vi "Set All Front Panel Controls Disabled State.vi"(8 "error in (no error)":errorcluster, 10 "Disabled":T1(ring), 11 "Actor in":refnum<class "Actor.lvclass">) -> (0 "error out":errorcluster, 3 "Actor out":refnum<class "Actor.lvclass">)   [LabVIEW 2015, in "Actor.lvclass"]
uses:
  Actor.lvclass
  Actor.lvclass/Actor.ctl
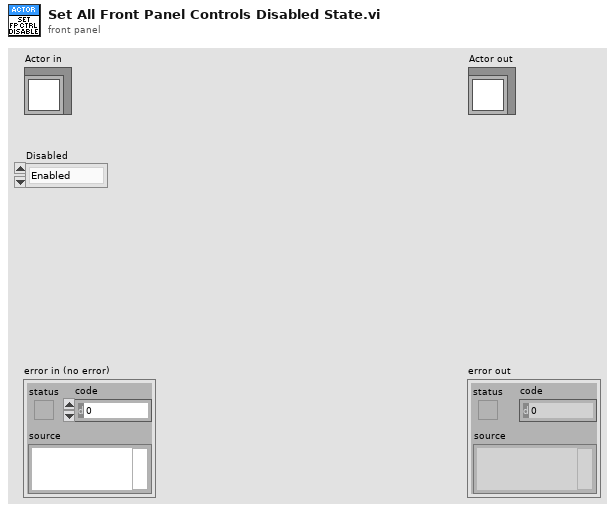
[diagram p1: front panel]
types:
  T1 = enum8{"Enabled", "Disabled", "Disabled and Grayed Out"}
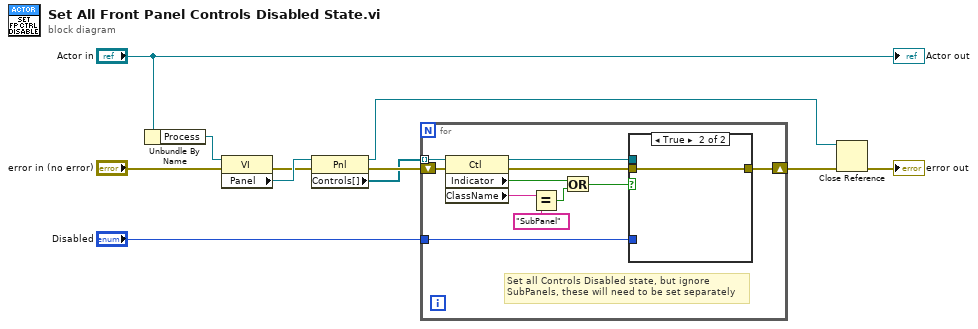
[diagram p0: block diagram]
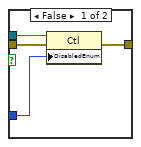
[diagram p2: hidden frame]
diagram:
  n1 = Unbundle By Name("Actor in") -> ("Process"=w6:refnum<vi>)
  n2 = property class="VI"(reference=w6, error in="error in (no error)") -> (error out=w10:errorcluster, "Panel"=w11:refnum<vi>)  [unwired: 1 out]
  n3 = property class="Pnl"(reference=w11, error in=w10) -> (reference out=w2:refnum<vi>, error out=w9:errorcluster, "Controls[]"=w1:refnum<vi>[])
  n4 = for {
    tunnel: w1 -> [w21] mode=indexing
    shift-right: [w17] -> w4
    shift-left: w9 -> [w20]
    tunnel: "Disabled" -> [w22]
    # "Set all Controls Disabled state, but ignore SubPanels, these will need to be set separately"
    n5 = property class="Ctl"(reference=w21, error in=w20) -> (reference out=w19:refnum<vi>, error out=w18:errorcluster, "Indicator"=w14:bool, "ClassName"=w16:string)
    n6 = Equal?(x=w16, y="SubPanel") -> (x = y?=w13:bool)
    n7 = Or(x=w14, y=w13) -> (x .or. y?=w12:bool)
    n8 = case shown="True" w12 {
      tunnel: w22 -> [w26 _]
      tunnel: w19 -> [w25 _]
      tunnel: w18 -> [w24 w27]
      tunnel: [w23 w27] -> w17
      frame False {
        n9 = property class="Ctl"(reference=w25, error in=w24, "DisabledEnum"=w26) -> (error out=w23:errorcluster)  [unwired: 1 out]
      }
      frame True {
      }
    }
  }
  n10 = Close Reference(reference=w2, error in (no error)=w4) -> (error out=→"error out":errorcluster)
  "Actor out" <- "Actor in"
